vi "testVoterRegistration.vi"(8 "error in (no error)":errorcluster, 11 "TestCase in":refnum<class "TestVoting.lvclass">) -> (0 "error out":errorcluster, 3 "TestCase out":refnum<class "TestVoting.lvclass">)   [LabVIEW 2019, in "TestVoting.lvclass"]
uses:
  TestVoting.lvclass
  <vilib>/addons/_JKI Toolkits/VI Tester/TestCase.llb/TestCase.lvclass
  C:/Program Files (x86)/National Instruments/LabVIEW 2019/vi.lib/addons/_JKI Toolkits/VI Tester/TestCase.llb/TestCase.lvclass
panel:
  out "map out":T1(c390)
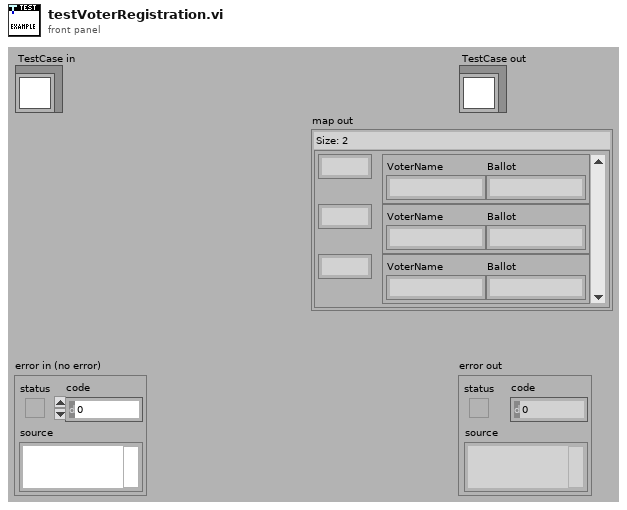
[diagram p1: front panel]
types:
  T1 = map{i32, cluster{"VoterName":string, "Ballot":string}}
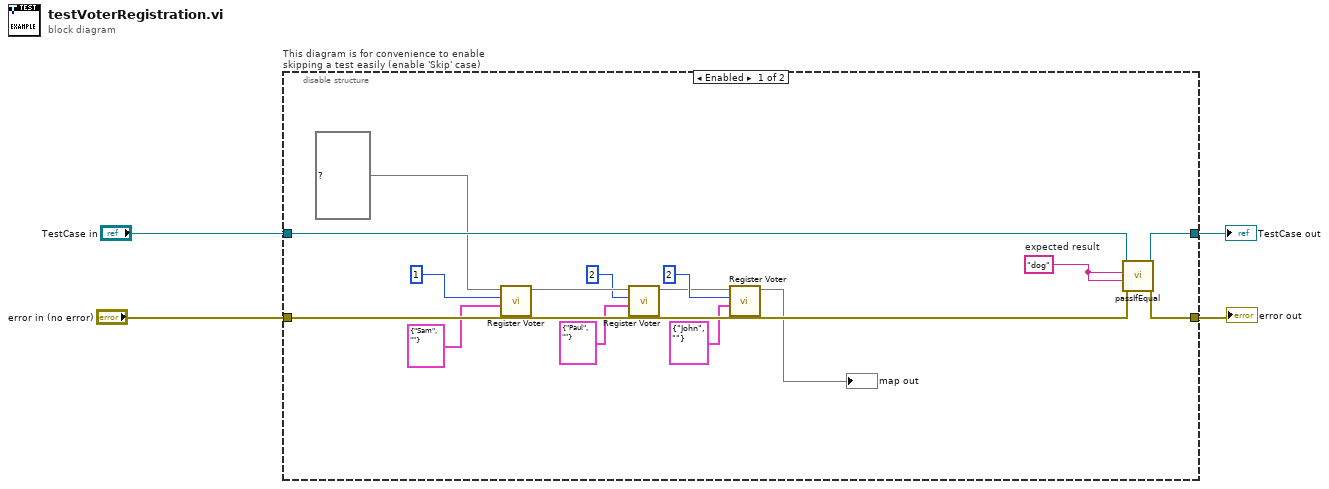
[diagram p0: block diagram]
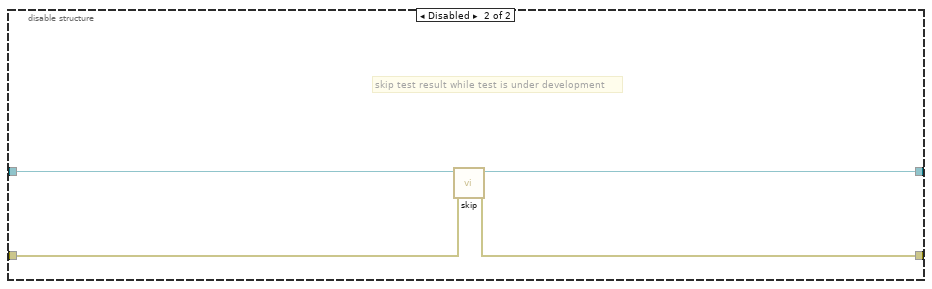
[diagram p2: hidden frame]
diagram:
  n1 = disable-structure "This diagram is for convenience to enable skipping a test easily (enable 'Skip' case)" shown="Enabled" {
    disable-tunnel: "TestCase in" -> [w19 w23]
    disable-tunnel: [w18 w21] -> w1
    disable-tunnel: [w17 w22] -> w3
    disable-tunnel: "error in (no error)" -> [w16 w20]
    frame Enabled {
      w9 = "dog"  # expected result
      n2 = call "Register Voter.vi"("VoterInfo"=cluster{"VoterName":string, "Ballot":string} {"VoterName"="Sam", "Ballot"=""}, "VoterID"=1, "map in"=T1 {} ("map")) -> ("map out"=w12:T1)  [unwired: 8 in]
      n3 = call "Register Voter.vi"("VoterInfo"=cluster{"VoterName":string, "Ballot":string} {"VoterName"="Paul", "Ballot"=""}, "VoterID"=2, "map in"=w12) -> ("map out"=w7:T1)  [unwired: 8 in]
      n4 = call "Register Voter.vi"("VoterInfo"=cluster{"VoterName":string, "Ballot":string} {"VoterName"="John", "Ballot"=""}, "VoterID"=2, "map in"=w7) -> ("map out"=→"map out":T1)  [unwired: 8 in]
      n5 = call-dynamic "passIfEqual.vi"("error in (no error)"=w16, "y"=w9, "x"=w9, "TestCase in"=w19) -> ("error out"=w17:errorcluster, "TestCase out"=w18:refnum<class "TestVoting.lvclass">)  [unwired: 6 in]
    }
    frame Disabled {
      # "skip test result while test is under development"
      n6 = call <vilib>:"skip.vi"("error in (no error)"=w20, "TestCase in"=w23) -> ("error out"=w22:errorcluster, "TestCase out"=w21:refnum<class "TestVoting.lvclass">)  [unwired: 8 in]
    }
  }
  "error out" <- w3
  "TestCase out" <- w1
